vi "Generate_in-collection_map.vi"(8 "error in (no error)":errorcluster, 9 "matched set":set{cluster{"CLZ ID":i32, "CV ID":i32}}(c389), 10 "CV Comics.lvclass":refnum<class "CV Comics.lvclass">, 11 "CLZ Comics.lvclass":refnum<class "CLZ Comics.lvclass">) -> (0 "error out":errorcluster)   [LabVIEW 2024, in "CLZ_to_ComicVine.lvlib"]
uses:
  CLZ_to_ComicVine.lvlib
  CLZ Comics/CLZ Comics.lvclass
  Volumes/CV Comics.lvclass
  CLZ Comics/CLZ Comics.lvclass/CLZ Comics.ctl
  CV_Shared_Library/CV_Shared_Library.lvlib
  <vilib>/addons/_JKI.lib/Serialization/JSON/JKI JSON Serialization.lvlib
panel:
  out "error probe":errorcluster
  out "Slide":u32(slide) scale=0.0..1626.0
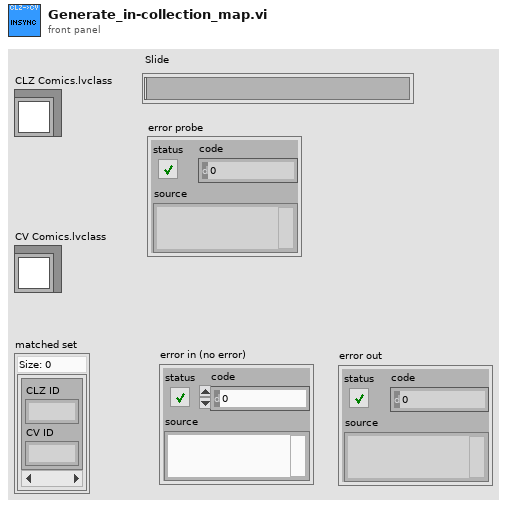
[diagram p1: front panel]
types:
  T1 = typedef "CLZ_to_ComicVine.lvlib/CLZ Comics.lvclass/volume--cluster.ctl" = cluster{"id":i32, "name":string, "issues":T2[], "matched":bool}
  T2 = typedef "CLZ_to_ComicVine.lvlib/CLZ Comics.lvclass/issue_number--cluster.ctl" = cluster{"numeric":dbl, "issue":string, "variant":string}
  T3 = typedef "CLZ_to_ComicVine.lvlib/issue_match--cluster.ctl" = cluster{"numeric":string, "issue":string, "id":string, "in clz":bool, "clz issue":T4}
  T4 = typedef "CLZ_to_ComicVine.lvlib/clz_matching_issue--cluster.ctl" = cluster{"numeric":string, "issue":string, "variant":string}
  T5 = typedef "CV_RESTful_Lib.lvlib/local_issue--cluster.ctl" = cluster{"cover_date":timestamp, "id":i32, "cv_id":string, "name":string, "sortable_name":string, "issue_number":string, "deck":string, "description":string, "volume":T6, "store_date":timestamp, "date_last_updated":timestamp, "site_detail_url":string, "cover_url":string, "associated_images":T7[], "characters":T6[], "concepts":T6[], "creators":T8[], "storyArcs":T6[], "teams":T6[], "in collection":bool}
  T6 = typedef "CV_RESTful_Lib.lvlib/cv_issue.generic_credit--cluster.ctl" = cluster{"id":i32, "name":string}
  T7 = typedef "CV_RESTful_Lib.lvlib/cv_issue.associated_image--cluster.ctl" = cluster{"original_url":string, "id":i32}
  T8 = typedef "CV_RESTful_Lib.lvlib/cv_issue.person_credit--cluster.ctl" = cluster{"id":i32, "name":string, "role":string}
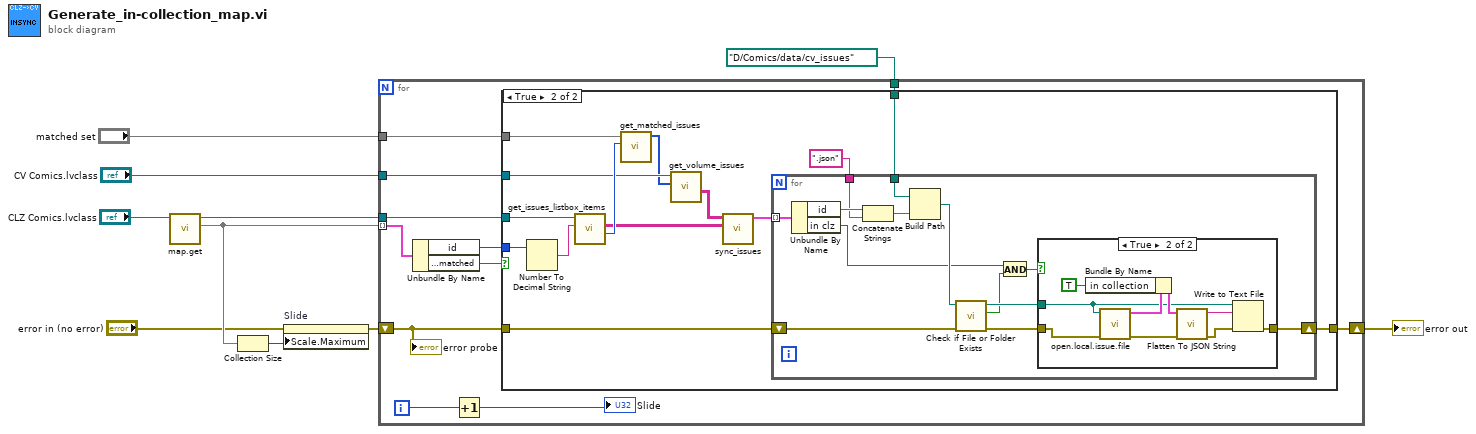
[diagram p0: block diagram]
diagram:
  n1 = call "map.get.vi"("CLZ Comics in"="CLZ Comics.lvclass") -> ("map"=w6:map{i32, T1}, "CLZ Comics out"=w9:refnum<class "CLZ Comics.lvclass">)  [unwired: 9 in]
  n2 = Collection Size(1:w6) -> (0:w5:i32)
  n3 = property on="Slide" class="Slide (strict)"(error in="error in (no error)", "Scale.Maximum"=w5) -> (error out=w4:errorcluster)  [unwired: 1 in, 1 out]
  n4 = for {
    tunnel: w6 -> [w19] mode=indexing
    tunnel: w9 -> [w18]
    tunnel: "matched set" -> [w17]
    tunnel: "CV Comics.lvclass" -> [w16]
    tunnel: path "D:/Comics/data/cv_issues" -> [w13]
    shift-right: [w12] -> w1
    shift-left: w4 -> [w11]
    i -> [w15]
    n5 = Unbundle By Name(w19) -> ("id"=w20:i32, "volume.matched"=w21:bool)
    n6 = Increment(x=w15) -> (x+1=→"Slide":i32)
    n7 = case shown="True" w21 {
      tunnel: w20 -> [_ w35]
      tunnel: w18 -> [_ w36]
      tunnel: w17 -> [_ w33]
      tunnel: w16 -> [_ w30]
      tunnel: w13 -> [_ w25]
      tunnel: w11 -> [w22 w24]
      tunnel: [w22 w23] -> w12
      frame False {
      }
      frame True {
        n8 = Number To Decimal String(number=w35) -> (decimal integer string=w34:string)  [unwired: 1 in]
        n9 = call "get_issues_listbox_items.vi"("CLZ Vol ID"=w34, "CLZ Comics in"=w36) -> ("id"=w32:i32, "listbox contents"=w31:string[][])  [unwired: 7 in, 1 out]
        n10 = call "get_matched_issues.vi"("id"=w32, "matched set"=w33) -> ("matched cv ids"=w28:i32[])  [unwired: 9 in]
        n11 = call "get_volume_issues.vi"("id"=w28, "CV Comics in"=w30) -> ("issues"=w29:string[][])  [unwired: 7 in, 2 out]
        n12 = call "sync_issues.vi"("CLZ Issues"=w31, "CV Issues"=w29) -> ("Array"=w27:T3[])  [unwired: 9 in]
        n13 = for {
          tunnel: w27 -> [w49] mode=indexing
          tunnel: ".json" ("string") -> [w47]
          tunnel: w25 -> [w45]
          shift-right: [w40] -> w23
          shift-left: w24 -> [w43]
          n14 = Unbundle By Name(w49) -> ("id"=w48:string, "in clz"=w39:bool)
          n15 = Concatenate Strings(w48, w47) -> (w46:string)
          n16 = Build Path(base path=w45, name or relative path=w46) -> (appended path=w44:path)
          n17 = call <vilib>:"Check if File or Folder Exists.vi"("error in (no error)"=w43, "path"=w44) -> ("error out"=w41:errorcluster, "file or folder exists?"=w38:bool, "dup path"=w42:path)  [unwired: 7 in]
          n18 = And(x=w39, y=w38) -> (x .and. y?=w37:bool)
          n19 = case shown="True" w37 {
            tunnel: w42 -> [_ w53]
            tunnel: w41 -> [w50 w59]
            tunnel: [w50 w52] -> w40
            frame False {
            }
            frame True {
              n20 = call "open.local.issue.file.vi"("error in (no error)"=w59, "issue json path"=w53) -> ("error out"=w55:errorcluster, "issue"=w56:T5)  [unwired: 8 in]
              n21 = Bundle By Name(cluster=w56, "in collection"=TRUE) -> (w54:T5)
              n22 = call <vilib>:"Flatten To JSON String.vi"("error in"=w55, "Variant"=w54) -> ("error out"=w58:errorcluster, "JSON String"=w57:string)  [unwired: 8 in]
              n23 = Write to Text File(file (use dialog)=w53, text=w57, error in=w58) -> (error out=w52:errorcluster)  [unwired: 1 in, 2 out]
            }
          }
        }
      }
    }
    "error probe" <- w11
  }
  "error out" <- w1
